vi "Parse-end-tag.vi"(6 "State data in":T1, 8 "error in (no error)":errorcluster, 10 "String in":string, 11 "Element-XML in":refnum<class "Element-XML.lvclass">) -> (0 "error out":errorcluster, 1 "Valid element?":bool, 2 "Remaining string":string, 3 "Element-XML out":refnum<class "Element-XML.lvclass">, 4 "State data":T1)   [LabVIEW 2013, in "MaterialCharacterization.lvlib" / "Element-XML.lvclass"]
uses:
  Element-XML.lvclass
  XML-parser-state.ctl
  Elements.ctl
  Element-XML.lvclass/Element-XML.ctl
  Write Parent ItemID.vi
  Write ItemID.vi
  Write Nesting level.vi
  Read Element.vi
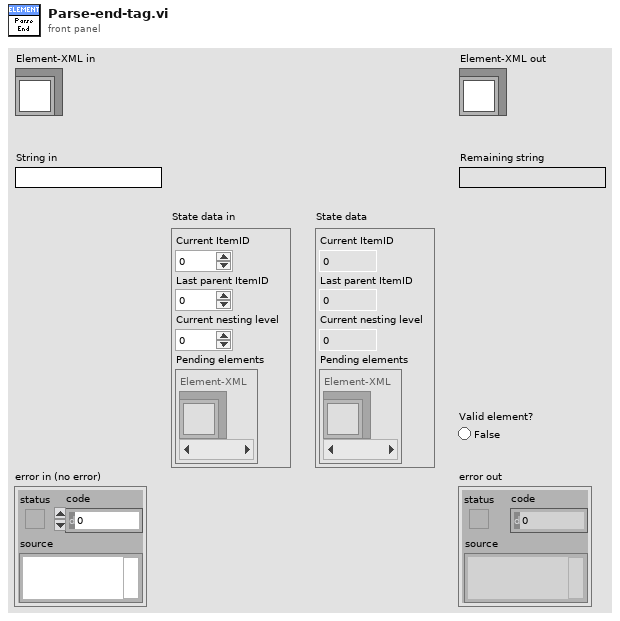
[diagram p1: front panel]
types:
  T1 = typedef "MaterialCharacterization.lvlib/Element-XML.lvclass/XML-parser-state.ctl" = cluster{"Current ItemID":u32, "Last parent ItemID":u32, "Current nesting level":i16, "Pending elements":refnum<class "Element-XML.lvclass">[]}
  T2 = typedef "MaterialCharacterization.lvlib/Element-XML.lvclass/Elements.ctl" = enum16{"BeginJob", "WriteDigital", "WriteAnalog", "Set", "ApplicationEvent", "JumpAbs", "MarkAbs", "JumpRel", "MarkRel", "LongDelay", "EndJob"}
  T3 = typedef "HardwareCharacterization.lvlib/Element-XML.lvclass/Elements.ctl" = enum16{"BeginJob", "WriteDigital", "WriteAnalog", "Set", "ApplicationEvent", "JumpAbs", "MarkAbs", "JumpRel", "MarkRel", "LongDelay", "EndJob"}
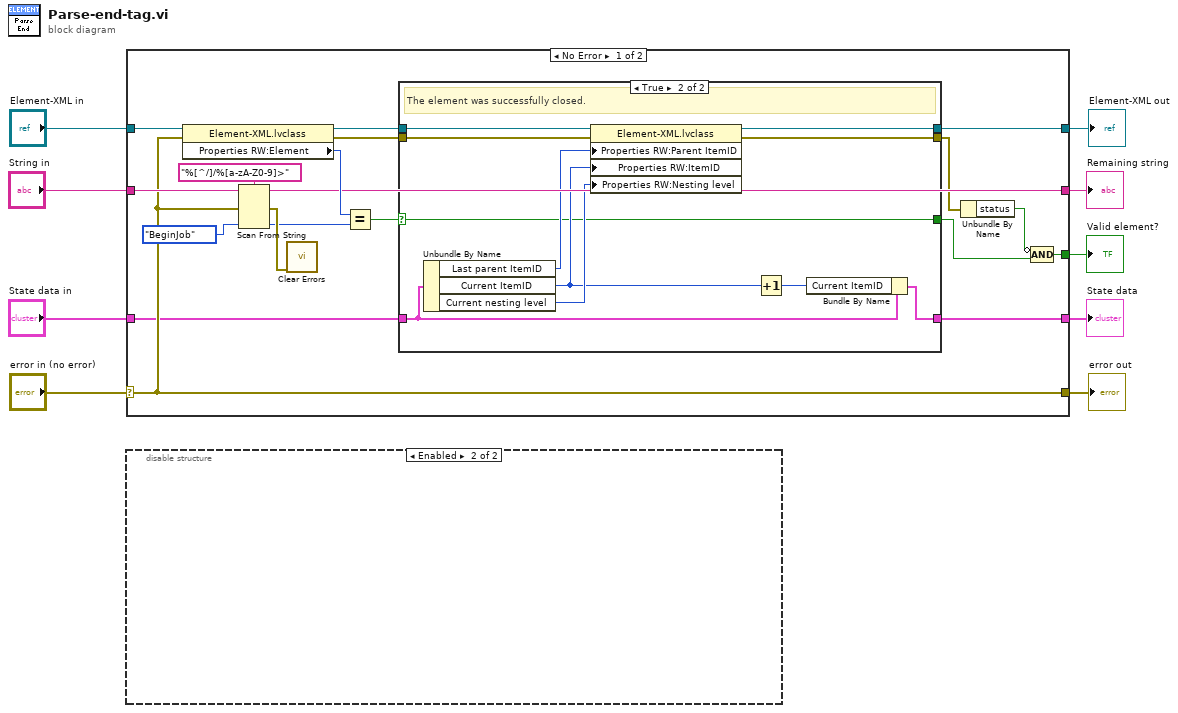
[diagram p0: block diagram]
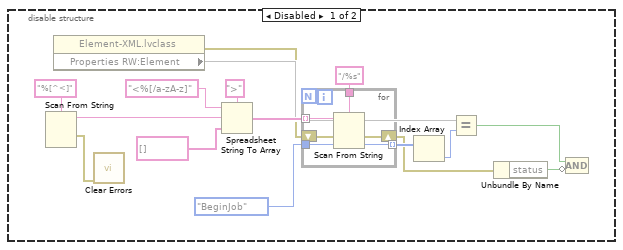
[diagram p2: hidden frame]
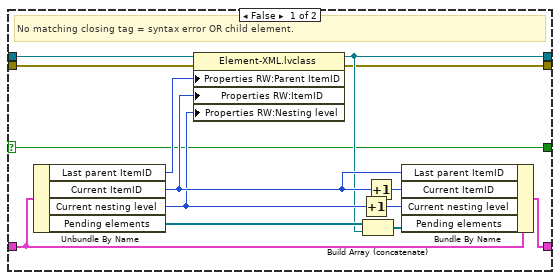
[diagram p3: hidden frame]
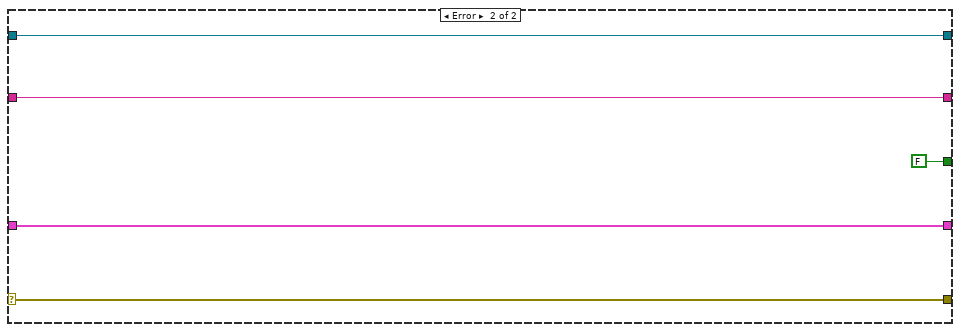
[diagram p4: hidden frame]
diagram:
  n1 = case shown="No Error" "error in (no error)" {
    selector: "error in (no error)" -> [w24 w58]
    tunnel: [w24 w58] -> w8
    tunnel: [w12 w57] -> w6
    tunnel: "Element-XML in" -> [w28 w57]
    tunnel: "String in" -> [w27 w54]
    tunnel: [w15 FALSE] -> w5
    tunnel: "State data in" -> [w19 w55]
    tunnel: [w18 w55] -> w3
    tunnel: [w20 w54] -> w1
    frame No Error {
      n2 = property class="Element-XML.lvclass"(reference=w28, error in=w24) -> (reference out=w14:refnum<class "Element-XML.lvclass">, error out=w13:errorcluster, "Properties RW:Element"=w21:T3)
      n3 = Scan From String(format string="%[^/]/%[a-zA-Z0-9]>", input string=w27, error in=w24, default 2=Elements."BeginJob" ("Element")) -> (remaining string=w20:string, error out=w25:errorcluster, output 2=w22:T2)  [unwired: 3 in, 1 out]
      n4 = call <vilib>:"Clear Errors.vi"("error in (no error)"=w25) -> ()  [unwired: 6 in, 1 out]
      n5 = Equal?(x=w21, y=w22) -> (x = y?=w16:bool)
      n6 = case shown="True" w16 {
        selector: w16 -> [w29 w43]
        tunnel: w19 -> [w42 w52]
        tunnel: [w41 w51] -> w18
        tunnel: w14 -> [w38 w50]
        tunnel: w13 -> [w31 w48]
        tunnel: [w32 w49] -> w12
        tunnel: [w30 w47] -> w11
        tunnel: [w29 w43] -> w10
        frame False {
          # "No matching closing tag = syntax error OR child element."
          n7 = Unbundle By Name(w42) -> ("Last parent ItemID"=w35:u32, "Current ItemID"=w34:u32, "Current nesting level"=w33:i16, "Pending elements"=w40:refnum<class "Element-XML.lvclass">[])
          n8 = property class="Element-XML.lvclass"(reference=w38, error in=w31, "Properties RW:Parent ItemID"=w35, "Properties RW:ItemID"=w34, "Properties RW:Nesting level"=w33) -> (reference out=w32:refnum<class "Element-XML.lvclass">, error out=w30:errorcluster)
          n9 = Increment(x=w33) -> (x+1=w37:i16)
          n10 = Build Array (concatenate)(w40, w32) -> (w39:refnum<class "Element-XML.lvclass">[])
          n11 = Increment(x=w34) -> (x+1=w36:u32)
          n12 = Bundle By Name(cluster=w42, "Last parent ItemID"=w34, "Current ItemID"=w36, "Current nesting level"=w37, "Pending elements"=w39) -> (w41:T1)
        }
        frame True {
          # "The element was successfully closed."
          n13 = Unbundle By Name(w52) -> ("Last parent ItemID"=w45:u32, "Current ItemID"=w44:u32, "Current nesting level"=w46:i16)
          n14 = property class="Element-XML.lvclass"(reference=w50, error in=w48, "Properties RW:Parent ItemID"=w45, "Properties RW:ItemID"=w44, "Properties RW:Nesting level"=w46) -> (reference out=w49:refnum<class "Element-XML.lvclass">, error out=w47:errorcluster)
          n15 = Increment(x=w44) -> (x+1=w53:u32)
          n16 = Bundle By Name(cluster=w52, "Current ItemID"=w53) -> (w51:T1)
        }
      }
      n17 = Unbundle By Name(w11) -> ("status"=w17:bool)
      n18 = Compound Arithmetic op=AND(invert w17, w10) -> (w15:bool)
    }
    frame Error {
    }
  }
  "error out" <- w8
  "Element-XML out" <- w6
  "Valid element?" <- w5
  "State data" <- w3
  "Remaining string" <- w1
  n19 = disable-structure shown="Enabled" {
    frame Disabled {
      n20 = Scan From String(format string="%[^<]") -> (remaining string=w69:string, error out=w73:errorcluster)  [unwired: 5 in, 1 out]
      n21 = property class="Element-XML.lvclass"() -> (error out=w63:errorcluster, "Properties RW:Element"=w65)  [unwired: 2 in, 1 out]
      n22 = call <vilib>:"Clear Errors.vi"("error in (no error)"=w73) -> ()  [unwired: 6 in, 1 out]
      n23 = Spreadsheet String To Array(delimiter (Tab)=">", format string="<%[/a-zA-z]", spreadsheet string=w69, array type (2D Dbl)=string[] []) -> (array=w68:string[])
      n24 = for {
        tunnel: w68 -> [w80] mode=indexing
        tunnel: Elements."BeginJob" ("Element") -> [w78]
        tunnel: [w77] -> w66 mode=indexing
        shift-right: [w76] -> w62
        shift-left: w63 -> [w79]
        tunnel: "/%s" -> [w75]
        n25 = Scan From String(format string=w75, input string=w80, error in=w79, default 1=w78) -> (error out=w76:errorcluster, output 1=w77:T2)  [unwired: 1 in, 2 out]
      }
      n26 = Index Array(array=w66) -> (element=w64:T2)  [unwired: 1 in]
      n27 = Equal?(x=w65, y=w64) -> (x = y?=w60:bool)
      n28 = Unbundle By Name(w62) -> ("status"=w61:bool)
      n29 = Compound Arithmetic op=AND(w60, invert w61) -> ()  [unwired: 1 out]
    }
    frame Enabled {
    }
  }
